vi "Stacked_Sequence.vi"   [LabVIEW 2017]
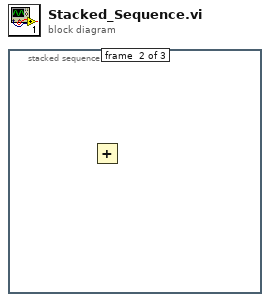
[diagram p0: block diagram]
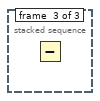
[diagram p3: hidden frame]
diagram:
  n1 = stacked-sequence {
    frame #0 {
    }
    frame #1 {
      n2 = Add() -> ()  [unwired: 2 in, 1 out]
    }
    frame #2 {
      n3 = Subtract() -> ()  [unwired: 2 in, 1 out]
    }
  }
